vi "U8ToFXP_Arrays.vi"(1 "Input":u8) -> (0 "Array":fxp<+/-,24,8>[](array[numeric]))   [LabVIEW 2018]
uses:
  <vilib>/rvi/Emulation/niFpgaSctlEmulationGetInTimedLoop.vi
  <vilib>/Utility/error.llb/Clear Errors.vi
  <vilib>/rvi/DataTransferAndStorage/Container/Common/niFpgaContainerGetUniqueNameForEmu.vi
  <vilib>/rvi/DataTransferAndStorage/Container/Common/niFpgaContainerSetEmuInfo.vi
  <vilib>/rvi/eio/common/nirviEmuReportErrorAndStop.vi
  <vilib>/rvi/DataTransferAndStorage/Container/Common/niFpgaContainerExecOnDevCompGetState.vi
  <vilib>/rvi/Emulation/niFpgaEmulationIsFPGAContextNoSignature.vi
  <vilib>/rvi/Emulation/niFpgaProcessEmulError.vi
  <vilib>/rvi/errors/nirviReportUnexpectedCaseInternalError (U32).vi
  <vilib>/rvi/Memory/Memory_Emulation/niFpgaMemoryEmulationCacheClearOnFirstRun.vi
  <vilib>/rvi/Memory/Memory_Emulation/nirvimemoryEmulationManagerCache_MakeExclusive.vi
  <vilib>/rvi/Memory/Memory_Emulation/niFpgaMemoryEmulationValidateCache.vi
  <vilib>/rvi/Memory/Memory_Emulation/nirvimemoryEmulationManagerCache_InsertValue.vi
  <vilib>/rvi/Memory/Memory_Emulation/nirvimemoryEmulationManagerCache_ReleaseExclusive.vi
  <vilib>/rvi/Memory/Memory_Emulation/nirvimemoryEmulationManagerCache_GetValue.vi
  <vilib>/rvi/Memory/Memory_Emulation/nirvimemoryEmulationManagerCache_SetValue.vi
  <vilib>/rvi/Emulation/niFpgaSctlEmulationResourceMgr.vi
  <vilib>/rvi/LocalResourceManager/LocalResourceManager.xnode
  <vilib>/rvi/DataTransferAndStorage/Container/XNode/niFpgaContainer.xnode
  <vilib>/rvi/Memory/Memory_Emulation/niFpgaMemoryEmulationRefIn.vi
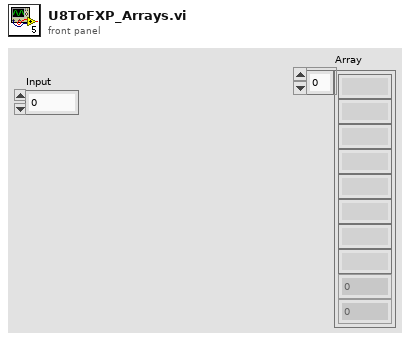
[diagram p1: front panel]
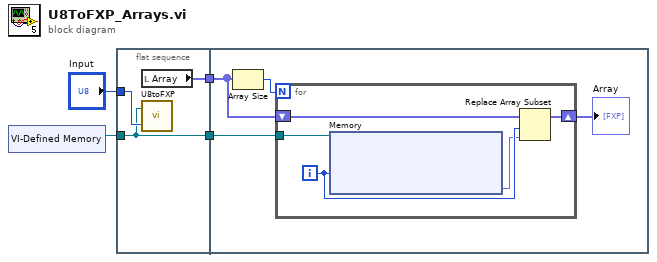
[diagram p0: block diagram]
diagram:
  n1 = xnode "VI-Defined Memory"() -> ("Memory Out"=w3:refnum<k21>)
  n2 = flat-sequence {
    tunnel: "Input" -> [w7]
    tunnel: w3 -> [w6]
    tunnel: [w6] -> w2
    tunnel: [w5] -> w1
    tunnel: w2 -> [w11]
    tunnel: w1 -> [w9]
    frame #0 {
      n3 = local read "Array"() -> (w5:fxp<+/-,24,8>[])
      n4 = call "U8toFXP.vi"("Input"=w7, "Values memory"=w6) -> ()  [unwired: 1 out]
    }
    frame #1 {
      n5 = Array Size(array=w9) -> (size(s)=w10:i32)
      n6 = for {
        N: w10 -> [_]
        tunnel: w11 -> [w14]
        shift-right: [w15] -> w8
        shift-left: w9 -> [w16]
        i -> [w13]
        n7 = xnode "Memory"("Address"=w13, "Memory In"=w14) -> ("Data"=w12:fxp<+/-,24,8>)  [unwired: 1 out]
        n8 = Replace Array Subset(array=w16, new element=w12, index=w13) -> (w15:fxp<+/-,24,8>[])
      }
      "Array" <- w8
    }
  }
